vi "WILT Shutdown All Valves.vi"(7 "Agilent Semaphore":T1[](array[typedef]), 8 "error in (no error)":errorcluster, 11 "Agilent Switches":T2[](array[typedef])) -> (0 "error out":errorcluster)   [LabVIEW 2016]
uses:
  Type Definitions/WILT Agilent Channel Definition.ctl
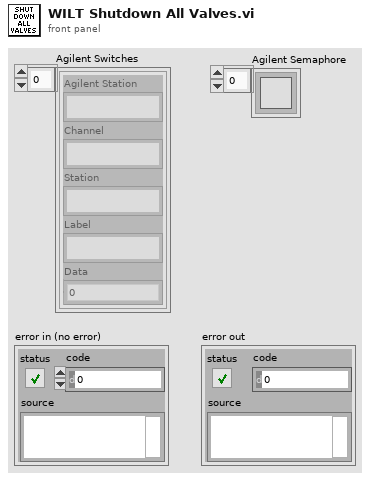
[diagram p1: front panel]
types:
  T1 = typedef "Semaphore RefNum" = refnum<k1>
  T2 = typedef "WILT Agilent Channel Definition.ctl" = cluster{"Channel":string, "Station":string, "Label":string, "Agilent Station":string, "Data":dbl}
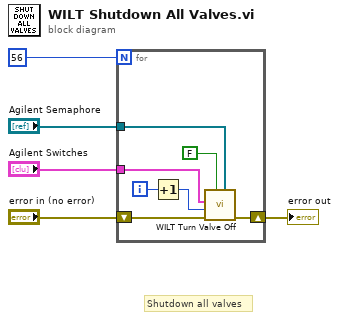
[diagram p0: block diagram]
diagram:
  # "Shutdown all valves"
  n1 = for {
    N: 56 -> [_]
    shift-right: [w6] -> w3
    shift-left: "error in (no error)" -> [w7]
    tunnel: "Agilent Switches" -> [w9]
    tunnel: "Agilent Semaphore" -> [w8]
    i -> [w11]
    n2 = Increment(x=w11) -> (x+1=w10:i32)
    n3 = call "WILT Turn Valve Off.vi"("Agilent Semaphore"=w8, "Remote Station"=FALSE, "Error In"=w7, "Station Index"=w10, "Agilent Valve and Switch Locations"=w9) -> ("Error Out"=w6:errorcluster)  [unwired: 6 in]
  }
  "error out" <- w3
